vi "sub_avi_codec.vi"(9 "Frames Per Second":u32=30, 10 "image array":T1[](array[typedef])) -> ()   [LabVIEW 2014]
uses:
  <vilib>/vision/Image Controls.llb/IMAQ Image.ctl
panel:
  out "segment byte array":u8[][](array[numeric])
  in  "codec index":i32
  out "codec":string
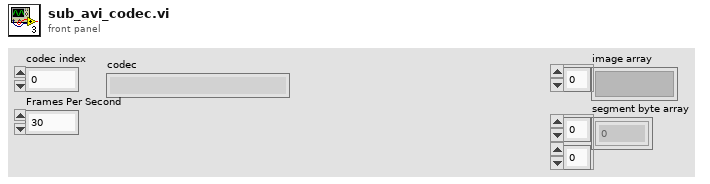
[diagram p1: front panel]
types:
  T1 = typedef "IMAQ Image.ctl" = refnum<image>
  T2 = typedef "IMAQ AVI2 Refnum.ctl" = refnum<k20>
  T3 = enum16{"open", "replace", "create", "open or create", "replace or create", "replace or create with confirmation"}
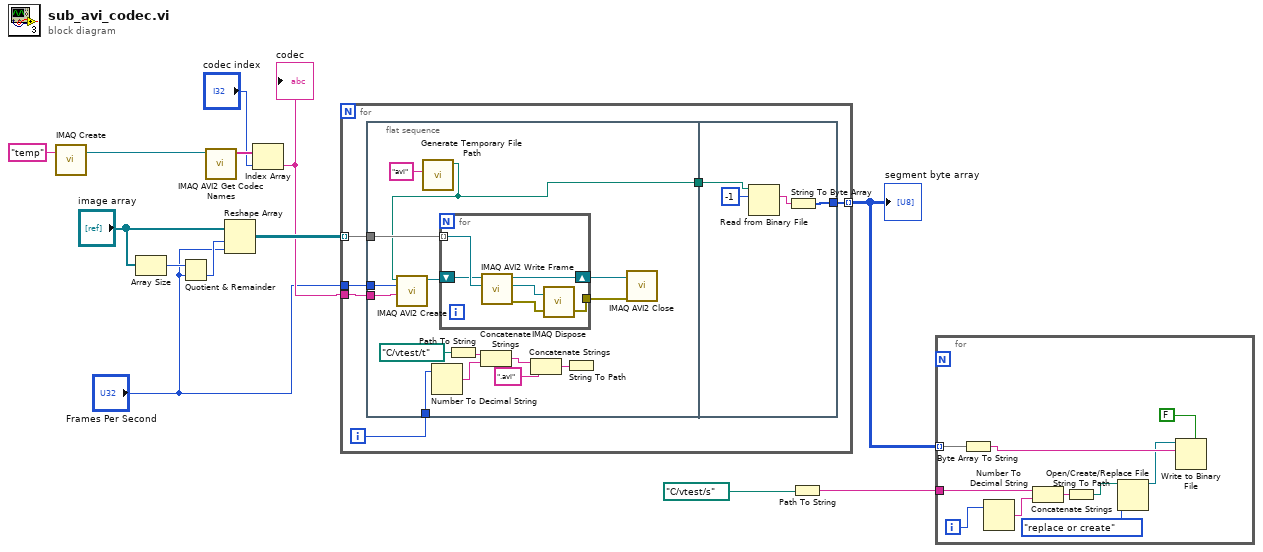
[diagram p0: block diagram]
diagram:
  n1 = call "IMAQ Create"("Image Name"="temp") -> ("New Image"=w9:T1)  [unwired: 4 in, 1 out]
  n2 = Array Size(array="image array") -> (size(s)=w13:i32)
  n3 = Quotient & Remainder(x=w13, y="Frames Per Second") -> (floor(x/y)=w2:u32)  [unwired: 1 out]
  n4 = call "IMAQ AVI2 Get Codec Names"("Image"=w9) -> ("Codec Names"=w11:string[])  [unwired: 9 in, 1 out]
  n5 = Reshape Array("image array", w2, "Frames Per Second") -> (w12:T1[][])
  n6 = Index Array(array=w11, index="codec index") -> (element=w3:string)
  "codec" <- w3
  n7 = for {
    tunnel: w12 -> [w19] mode=indexing
    tunnel: [w18] -> w6 mode=indexing
    tunnel: w3 -> [w16]
    tunnel: "Frames Per Second" -> [w17]
    i -> [w15]
    n8 = flat-sequence {
      tunnel: w19 -> [w34]
      tunnel: w17 -> [w33]
      tunnel: w16 -> [w32]
      tunnel: w15 -> [w27]
      tunnel: [w20] -> w14
      tunnel: [w43] -> w18
      tunnel: w14 -> [w41]
      frame #0 {
        n9 = call <vilib>:"Generate Temporary File Path.vi"("Temporary File Extension (tmp)"="avi") -> ("Unique Temporary File Path"=w20:path)  [unwired: 9 in, 1 out]
        n10 = call "IMAQ AVI2 Create"("Codec"=w32, "Frames Per Second"=w33, "AVI Path"=w20) -> ("AVI Refnum"=w30:T2)  [unwired: 7 in, 1 out]
        n11 = Number To Decimal String(number=w27) -> (decimal integer string=w28:string)  [unwired: 1 in]
        n12 = for {
          tunnel: w34 -> [w40] mode=indexing
          shift-right: [w37] -> w21
          shift-left: w30 -> [w36]
          tunnel: [w35] -> w29
          n13 = call "IMAQ AVI2 Write Frame"("Image"=w40, "AVI Refnum"=w36) -> ("error out"=w38:errorcluster, "Image Out (duplicate)"=w39:T1, "AVI Refnum (duplicate)"=w37:T2)  [unwired: 7 in]
          n14 = call "IMAQ Dispose"("Image"=w39, "error in (no error)"=w38) -> ("error out"=w35:errorcluster)  [unwired: 4 in]
        }
        n15 = Path To String(path=path "C:/vtest/t" ("file (use dialog)")) -> (string=w25:string)
        n16 = Concatenate Strings(w25, w28) -> (w24:string)
        n17 = Concatenate Strings(w24, ".avi" ("string")) -> (w22:string)
        n18 = String To Path(string=w22) -> ()  [unwired: 1 out]
        n19 = call "IMAQ AVI2 Close"("error in (no error)"=w29, "AVI Refnum"=w21) -> ()  [unwired: 9 in, 1 out]
      }
      frame #1 {
        n20 = Read from Binary File(10:-1 ("count (1)"), 11:w41) -> (2:w44:string)  [unwired: 4 in, 3 out]
        n21 = String To Byte Array(string=w44) -> (unsigned byte array=w43:u8[])
      }
    }
  }
  "segment byte array" <- w6
  n22 = Path To String(path=path "C:/vtest/s" ("file (use dialog)")) -> (string=w4:string)
  n23 = for {
    tunnel: w6 -> [w54] mode=indexing
    tunnel: w4 -> [w50]
    i -> [w52]
    n24 = Byte Array To String(unsigned byte array=w54) -> (string=w53:string)
    n25 = Number To Decimal String(number=w52) -> (decimal integer string=w51:string)  [unwired: 1 in]
    n26 = Concatenate Strings(w50, w51) -> (w49:string)
    n27 = String To Path(string=w49) -> (path=w48:path)
    n28 = Open/Create/Replace File(file path (use dialog)=w48, operation (0:open)=T3."replace or create") -> (refnum out=w47:refnum<file>)  [unwired: 4 in, 2 out]
    n29 = Write to Binary File(file (use dialog)=w47, data=w53, 5:FALSE ("prepend array or string size? (T)")) -> ()  [unwired: 3 in, 3 out]
  }
